vi "Measurement.Free.UI.SetDependencies.vi"(8 "error in (no error)":errorcluster, 10 "Dependencies":T1, 11 "Measurement.Free.UI in":refnum<class "Measurement.Free.UI.lvclass">) -> (0 "error out":errorcluster, 3 "Measurement.Free.UI out":refnum<class "Measurement.Free.UI.lvclass">)   [LabVIEW 2019, in "Measurement.Free.UI.lvclass"]
uses:
  Measurement.Free.UI.lvclass
  Typedefs/Dependencies--Cluster.ctl
  Measurement.Free/Measurement.Free.lvclass
  Measurement.Free.UI.lvclass/Measurement.Free.UI.ctl
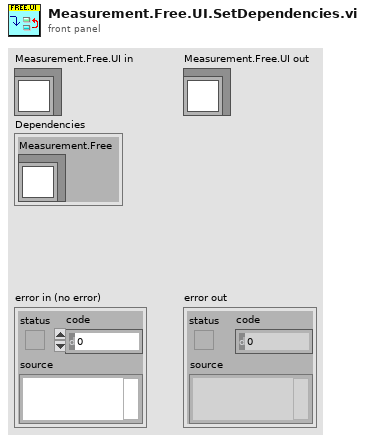
[diagram p1: front panel]
types:
  T1 = typedef "Measurement.Free.UI.lvclass/Dependencies--Cluster.ctl" = cluster{"Measurement.Free":refnum<class "Measurement.Free.lvclass">}
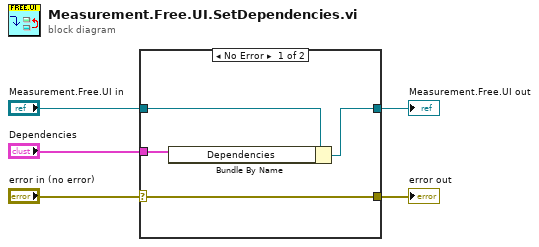
[diagram p0: block diagram]
diagram:
  n1 = case shown="No Error" "error in (no error)" {
    selector: "error in (no error)" -> [w9 w11]
    tunnel: [w9 w11] -> w4
    tunnel: [w6 w10] -> w2
    tunnel: "Measurement.Free.UI in" -> [w8 w10]
    tunnel: "Dependencies" -> [w7 _]
    frame No Error {
      n2 = Bundle By Name(cluster=w8, "Dependencies"=w7) -> (w6:refnum<class "Measurement.Free.UI.lvclass">)
    }
    frame Error {
    }
  }
  "error out" <- w4
  "Measurement.Free.UI out" <- w2
